vi "子VI-查看某框.vi"(0 "输入框号（默认值0为整张图）":dbl format="%#_13g", 1 "框组":T3(array[cluster]), 2 "临界Z值":i32, 3 "反射图原始路径":path, 4 "临界面积百分比值":dbl, 5 "预先配置的灰度阈值":dbl, 6 "穿透图原始路径":path, 7 "部位信息":string[](array[string])=["", "34.500000", "32.500000", "1121", "34", "54.955926", "分层类", "不合格", ""], 12 "产品规格":cluster{"产品长度（周长）（mm）":dbl, "产品宽度（母线长）（mm）":dbl}) -> (14 "全部检测结果":string[][](table))   [LabVIEW 2018]
uses:
  <vilib>/vision/NI_Vision_Development_Module.lvlib
panel:
  out "弥散类检测结果":string[][](table)
  out "?":string[][](table)
  in  "格式字符串 4":string="%f"
  in  "分隔符（'\\'代码显示） 3":string="\t"
  in  "返回主界面":bool caption="辅助定性分析"
  in  "格式字符串 3":string="%f"
  in  "分隔符（'\\'代码显示） 2":string="\t"
  out "弥散缺陷个数":i32
  out "分层缺陷个数":i32
  out "合格？ 弥散类":string="fencengThreshold"
  out "合格？分层类":string="fencengThreshold"
  in  "Tab Control":T1
  out "穿透ROI":T2(plugin-control)
  out "Threshold Image":T2(plugin-control)
  out "?":T2(plugin-control)
  out "?":T2(plugin-control)
  out "Threshold Image":T2(plugin-control)
  out "Threshold Image":T2(plugin-control)
  out "弥散测量结果":dbl[][](array[numeric]) format="%.2f"
  out "?":string
  out "面积 (pixels)":i32
  in  "格式字符串 2":string="%f"
  in  "分隔符（'\\'代码显示）":string="\t"
  out "分层测量结果":dbl[][](array[numeric]) format="%.2f"
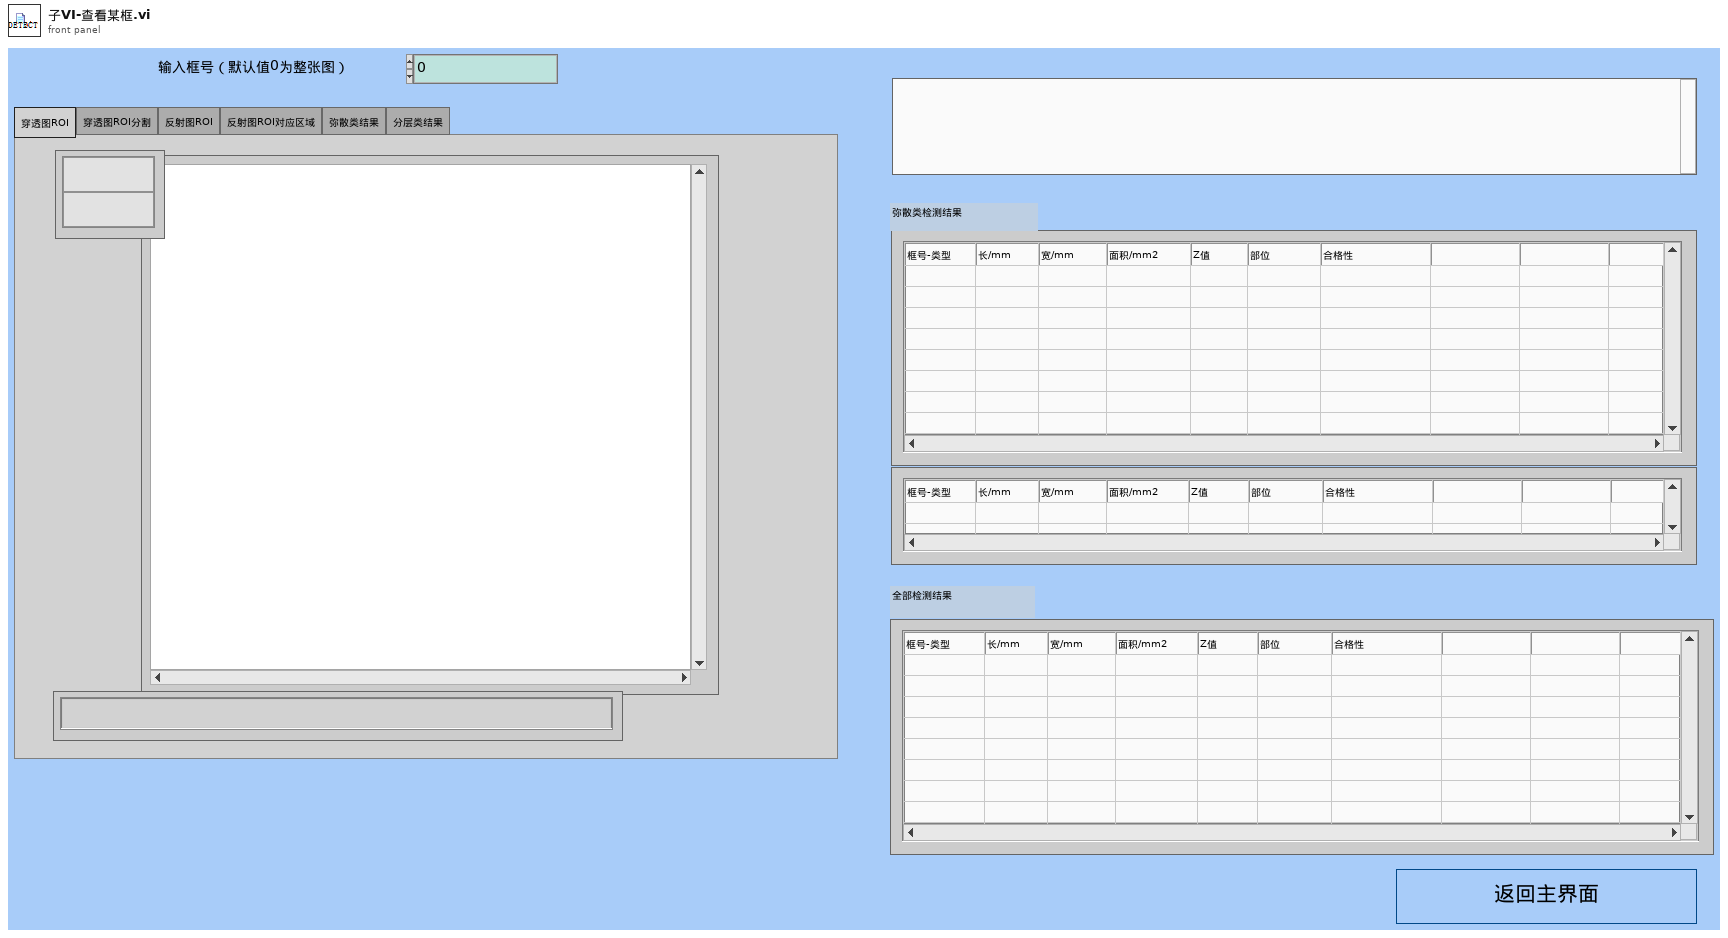
[diagram p1: front panel]
types:
  T1 = typedef "控件 1.ctl" = enum32{"穿透图ROI", "穿透图ROI分割", "反射图ROI", "反射图ROI对应区域", "弥散类结果", "分层类结果"}
  T2 = typedef "IMAQ Image.ctl" = refnum<image>
  T3 = cluster{"Global Rectangle":i32[], "Contours":cluster{"Contour Type":u32, "ROI Type":u32, "Points":i32[]}[]}[]
  T4 = cluster{"Zoom Tool":bool, "Selection Tool":bool, "Pan Tool":bool, "Point Tool":bool, "Line Tool":bool, "Rectangle Tool":bool, "Rotated Rectangle Tool":bool, "Polyline Tool":bool, "Polygon Tool":bool, "Freehand Tool":bool, "Closed Freehand Tool":bool, "Ellipse Tool":bool, "Annulus Tool":bool}
  T5 = typedef "Image Type" = u32
  T6 = typedef "Particle Parameters" = i32
  T7 = cluster{"Measurement Parameter":T6, "Range Lower Value":dbl, "Range Upper Value":dbl, "Range":bool, "Measurement Type":bool}[]
  T8 = cluster{"Global Rectangle":i32[], "Contours":cluster{"Contour Type":u32, "ROI Type":u32, "Points":i32[]}[]}
  T9 = cluster{"histogram":u32[], "Minimal Value":sgl, "Maximal Value":sgl, "Starting Value":sgl, "Interval Width":sgl, "Mean Value":sgl, "Standard  Variation":sgl, "Area (pixels)":i32}
  T10 = cluster{"Area":dbl, "Number of Holes":dbl, "Bounding Rect":cluster{"Left":dbl, "Top":dbl, "Right":dbl, "Bottom":dbl}, "Center of Mass":cluster{"X":dbl, "Y":dbl}, "Orientation":dbl, "Dimensions":cluster{"Width":dbl, "Height":dbl}}[]
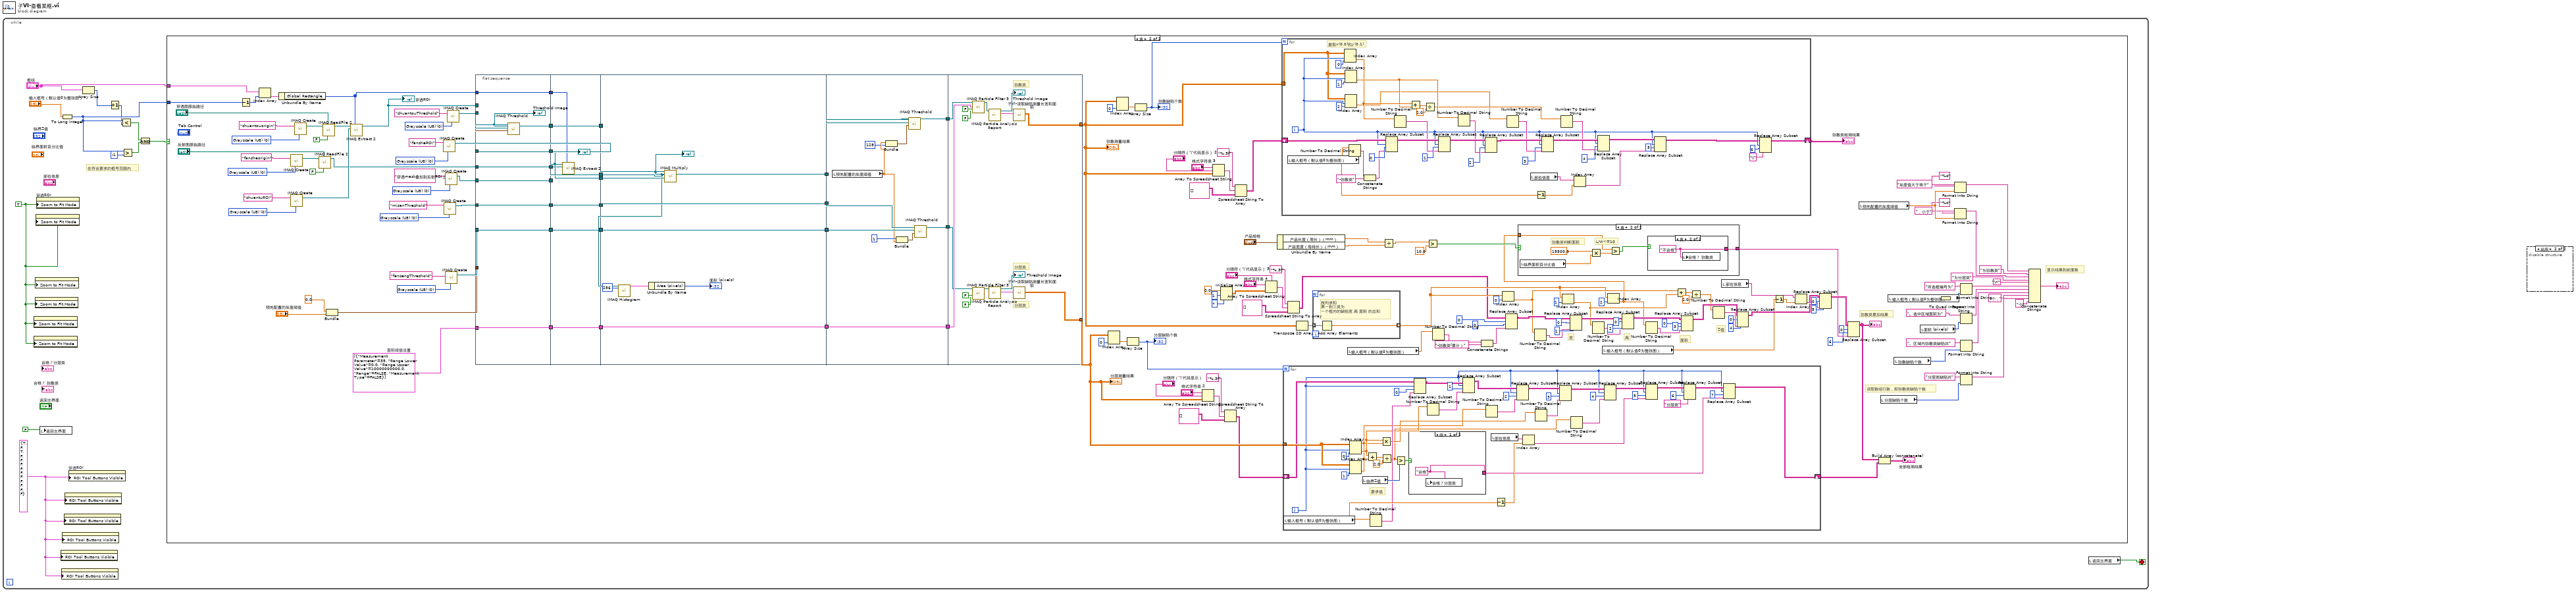
[diagram p0: block diagram]
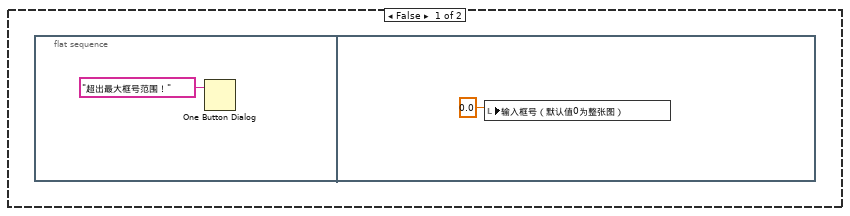
[diagram p2: hidden frame]
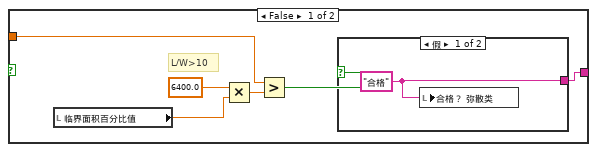
[diagram p3: hidden frame]
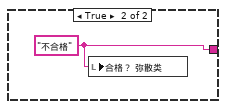
[diagram p4: hidden frame]
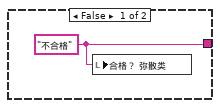
[diagram p5: hidden frame]
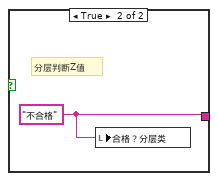
[diagram p6: hidden frame]
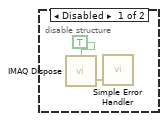
[diagram p7: hidden frame]
diagram:
  n1 = while {
    stop <- w5 stop-if-true
    w3 = T4 {"Zoom Tool"=TRUE, "Selection Tool"=FALSE, "Pan Tool"=TRUE, "Point Tool"=FALSE, "Line Tool"=FALSE, "Rectangle Tool"=FALSE, "Rotated Rectangle Tool"=FALSE, "Polyline Tool"=FALSE, "Polygon Tool"=FALSE, "Freehand Tool"=FALSE, "Closed Freehand Tool"=FALSE, "Ellipse Tool"=FALSE, "Annulus Tool"=FALSE} ("ROI Tool Buttons Visible:All Elements")
    w13 = TRUE ("Zoom to Fit Mode")
    # "在符合要求的框号范围内"
    n2 = property class="ImageControl"("Zoom to Fit Mode"=w13) -> ()  [unwired: 2 in, 2 out]
    n3 = property class="ImageControl"("Zoom to Fit Mode"=w13) -> ()  [unwired: 2 in, 2 out]
    n4 = property class="ImageControl"("Zoom to Fit Mode"=w13) -> ()  [unwired: 2 in, 2 out]
    n5 = property class="ImageControl"("Zoom to Fit Mode"=w13) -> ()  [unwired: 2 in, 2 out]
    n6 = property class="ImageControl"("Zoom to Fit Mode"=w13) -> ()  [unwired: 2 in, 2 out]
    n7 = property on="穿透ROI" class="ImageControl"("Zoom to Fit Mode"=w13) -> ()  [unwired: 2 in, 2 out]
    n8 = local write "返回主界面"(FALSE ("stop")) -> ()
    n9 = property class="ImageControl"("ROI Tool Buttons Visible"=w3) -> ()  [unwired: 2 in, 2 out]
    n10 = To Long Integer(number="输入框号（默认值0为整张图）") -> (32bit integer=w6:i32)
    n11 = property class="ImageControl"("ROI Tool Buttons Visible"=w3) -> ()  [unwired: 2 in, 2 out]
    n12 = property class="ImageControl"("ROI Tool Buttons Visible"=w3) -> ()  [unwired: 2 in, 2 out]
    n13 = property class="ImageControl"("ROI Tool Buttons Visible"=w3) -> ()  [unwired: 2 in, 2 out]
    n14 = property class="ImageControl"("ROI Tool Buttons Visible"=w3) -> ()  [unwired: 2 in, 2 out]
    n15 = property on="穿透ROI" class="ImageControl"("ROI Tool Buttons Visible"=w3) -> ()  [unwired: 2 in, 2 out]
    n16 = Array Size(array="框组") -> (size(s)=w2:i32)
    n17 = Increment(x=w2) -> (x+1=w1:i32)
    n18 = Less?(x=w6, y=w1) -> (x < y?=w11:bool)
    n19 = Greater?(x=w6, y=-1) -> (0:w10:bool)
    n20 = And(x=w11, y=w10) -> (x .and. y?=w4:bool)
    n21 = case shown="真" w4 {
      tunnel: "框组" -> [_ w77]
      tunnel: w6 -> [_ w76]
      frame False {
        n22 = flat-sequence {
          frame #0 {
            n23 = One Button Dialog(message="超出最大框号范围！" ("消息")) -> ()  [unwired: 1 in, 1 out]
          }
          frame #1 {
            n24 = local write "输入框号（默认值0为整张图）"(0.0 ("框号")) -> ()
          }
        }
      }
      frame True {
        w135 = T5 0 items=["Grayscale (U8)", "Grayscale (I16)", "Grayscale (SGL)", "Complex (CSG)", "RGB (U32)", "HSL (U32)", "RGB (U64)", "Grayscale (U16)"] ("Image Type")
        w136 = T5 0 items=["Grayscale (U8)", "Grayscale (I16)", "Grayscale (SGL)", "Complex (CSG)", "RGB (U32)", "HSL (U32)", "RGB (U64)", "Grayscale (U16)"] ("Image Type")
        w137 = T5 0 items=["Grayscale (U8)", "Grayscale (I16)", "Grayscale (SGL)", "Complex (CSG)", "RGB (U32)", "HSL (U32)", "RGB (U64)", "Grayscale (U16)"] ("Image Type")
        w141 = T5 0 items=["Grayscale (U8)", "Grayscale (I16)", "Grayscale (SGL)", "Complex (CSG)", "RGB (U32)", "HSL (U32)", "RGB (U64)", "Grayscale (U16)"] ("Image Type")
        w145 = T5 0 items=["Grayscale (U8)", "Grayscale (I16)", "Grayscale (SGL)", "Complex (CSG)", "RGB (U32)", "HSL (U32)", "RGB (U64)", "Grayscale (U16)"] ("Image Type")
        w120 = T7 [{"Measurement Parameter"=35, "Range Lower Value"=0.0, "Range Upper Value"=10000000000.0, "Range"=FALSE, "Measurement Type"=FALSE}]  # 面积阈值设置
        w156 = T5 0 items=["Grayscale (U8)", "Grayscale (I16)", "Grayscale (SGL)", "Complex (CSG)", "RGB (U32)", "HSL (U32)", "RGB (U64)", "Grayscale (U16)"] ("Image Type")
        w129 = T5 0 items=["Grayscale (U8)", "Grayscale (I16)", "Grayscale (SGL)", "Complex (CSG)", "RGB (U32)", "HSL (U32)", "RGB (U64)", "Grayscale (U16)"] ("Image Type")
        w160 = T5 0 items=["Grayscale (U8)", "Grayscale (I16)", "Grayscale (SGL)", "Complex (CSG)", "RGB (U32)", "HSL (U32)", "RGB (U64)", "Grayscale (U16)"] ("Image Type")
        # "弥散类累加结果"
        # "Z值"
        # "面积"
        # "高"
        # "宽"
        # "显示结果到前面板"
        # "读取数组行数，即弥散类缺陷个数"
        n25 = Decrement(x=w76) -> (x-1=w162:i32)
        n26 = Index Array(array=w77, index=w162) -> (element=w163:T8)
        n27 = Unbundle By Name(w163) -> ("Global Rectangle"=w128:i32[])
        n28 = call "IMAQ Create"("Image Name"="fansheorigin", "Image Type"=w141) -> ("New Image"=w140:T2)  [unwired: 3 in, 1 out]
        n29 = call "IMAQ Create"("Image Name"="chuantuROI", "Image Type"=w145) -> ("New Image"=w144:T2)  [unwired: 3 in, 1 out]
        n30 = call "IMAQ Create"("Image Name"="chuantouorigin", "Image Type"=w160) -> ("New Image"=w147:T2)  [unwired: 3 in, 1 out]
        n31 = call "IMAQ ReadFile 2"("Use File Path Image Type"=FALSE, "File Path"="反射图原始路径", "Image"=w140) -> ("Image Out"=w124:T2)  [unwired: 4 in, 4 out]
        n32 = call "IMAQ ReadFile 2"("Use File Path Image Type"=FALSE, "File Path"="穿透图原始路径", "Image"=w147) -> ("Image Out"=w148:T2)  [unwired: 4 in, 4 out]
        n33 = Bundle(0.0, "预先配置的灰度阈值"="预先配置的灰度阈值") -> (w119:cluster{dbl, "预先配置的灰度阈值":dbl})  [unwired: 1 in]
        n34 = call "IMAQ Extract 2"("Optional Rectangle"=w128, "Image Dst"=w144, "Image Src"=w148) -> ("Image Dst Out"=w126:T2)  [unwired: 7 in, 1 out]
        "穿透ROI" <- w126
        n35 = call "IMAQ Create"("Image Name"="fansheROI", "Image Type"=w129) -> ("New Image"=w125:T2)  [unwired: 3 in, 1 out]
        n36 = call "IMAQ Create"("Image Name"="misanThreshold", "Image Type"=w135) -> ("New Image"=w122:T2)  [unwired: 3 in, 1 out]
        n37 = call "IMAQ Create"("Image Name"="穿透mask叠加到反射ROI上", "Image Type"=w156) -> ("New Image"=w123:T2)  [unwired: 3 in, 1 out]
        n38 = call "IMAQ Create"("Image Name"="fencengThreshold", "Image Type"=w136) -> ("New Image"=w121:T2)  [unwired: 3 in, 1 out]
        n39 = call "IMAQ Create"("Image Name"="chuantouThreshold", "Image Type"=w137) -> ("New Image"=w127:T2)  [unwired: 3 in, 1 out]
        n40 = flat-sequence {
          tunnel: w128 -> [w257]
          tunnel: w127 -> [w256]
          tunnel: w126 -> [w255]
          tunnel: w119 -> [w254]
          tunnel: w125 -> [w253]
          tunnel: w124 -> [w252]
          tunnel: [w257] -> w186
          tunnel: [w253] -> w185
          tunnel: [w252] -> w184
          tunnel: [w251] -> w183
          tunnel: w123 -> [w251]
          tunnel: [w250] -> w182
          tunnel: w122 -> [w249]
          tunnel: [w249] -> w181
          tunnel: [w248] -> w180
          tunnel: w121 -> [w248]
          tunnel: [w247] -> w179
          tunnel: w120 -> [w247]
          tunnel: w186 -> [w266]
          tunnel: w185 -> [w258]
          tunnel: w184 -> [w259]
          tunnel: w183 -> [w265]
          tunnel: [w265] -> w178
          tunnel: [w264] -> w177
          tunnel: w182 -> [w264]
          tunnel: [w263] -> w176
          tunnel: w181 -> [w262]
          tunnel: [w262] -> w175
          tunnel: w180 -> [w261]
          tunnel: [w261] -> w174
          tunnel: w179 -> [w260]
          tunnel: [w260] -> w173
          tunnel: w178 -> [w276]
          tunnel: w177 -> [w275]
          tunnel: w176 -> [w274]
          tunnel: [w273] -> w172
          tunnel: w175 -> [w273]
          tunnel: w174 -> [w272]
          tunnel: [w272] -> w171
          tunnel: [w268] -> w170
          tunnel: w173 -> [w267]
          tunnel: [w267] -> w169
          tunnel: w172 -> [w287]
          tunnel: w171 -> [w286]
          tunnel: w170 -> [w285]
          tunnel: [w284] -> w168
          tunnel: [w283] -> w167
          tunnel: w169 -> [w282]
          tunnel: [w282] -> w166
          tunnel: [w291] -> w65
          tunnel: [w294] -> w108
          tunnel: w168 -> [w297]
          tunnel: w167 -> [w296]
          tunnel: w166 -> [w300]
          frame #0 {
            n41 = call "IMAQ Threshold"("Range"=w254, "Image Dst"=w256, "Image Src"=w255) -> ("Image Dst Out"=w250:T2)  [unwired: 3 in, 5 out]
            "Threshold Image" <- w250
          }
          frame #1 {
            n42 = call "IMAQ Extract 2"("Optional Rectangle"=w266, "Image Dst"=w258, "Image Src"=w259) -> ("Image Dst Out"=w263:T2)  [unwired: 7 in, 1 out]
            "?" <- w263
          }
          frame #2 {
            n43 = call "IMAQ Multiply"("Image Src A"=w275, "Image Dst"=w276, "Image Src B"=w274) -> ("Image Dst Out"=w268:T2)  [unwired: 4 in, 1 out]
            "?" <- w268
            n44 = call "IMAQ Histogram"("Number of Classes"=256, "Image"=w268) -> ("Histogram Report"=w270:T9)  [unwired: 8 in, 1 out]
            n45 = Unbundle By Name(w270) -> ("Area (pixels)"=→"面积 (pixels)":i32)
          }
          frame #3 {
            n46 = local read "预先配置的灰度阈值"() -> (w278:dbl)
            n47 = Bundle("预先配置的灰度阈值"=w278, 128) -> (w281:cluster{"预先配置的灰度阈值":dbl, i32})  [unwired: 1 in]
            n48 = Bundle(1, "预先配置的灰度阈值"=w278) -> (w280:cluster{i32, "预先配置的灰度阈值":dbl})  [unwired: 1 in]
            n49 = call "IMAQ Threshold"("Range"=w281, "Image Dst"=w287, "Image Src"=w285) -> ("Image Dst Out"=w283:T2)  [unwired: 3 in, 5 out]
            n50 = call "IMAQ Threshold"("Range"=w280, "Image Dst"=w286, "Image Src"=w285) -> ("Image Dst Out"=w284:T2)  [unwired: 3 in, 5 out]
          }
          frame #4 {
            # "分层类"
            # "分层类"
            # "弥散类"
            n51 = call "IMAQ Particle Filter 3"("Image Src"=w296, "Selection Values"=w300, "Keep/Remove Particles (F)"=FALSE, "Reject Border? (F)"=FALSE) -> ("Image Dst Out"=w289:T2)  [unwired: 9 in, 2 out]
            n52 = call "IMAQ Particle Filter 3"("Image Src"=w297, "Keep/Remove Particles (F)"=FALSE, "Reject Border? (F)"=FALSE) -> ("Image Dst Out"=w292:T2)  [unwired: 10 in, 2 out]
            n53 = call "IMAQ Particle Analysis Report"("Image"=w289) -> ("Particle Reports (Pixels)"=w290:T10, "Image Out (duplicate)"=→"Threshold Image":T2)  [unwired: 5 in, 4 out]
            n54 = call "IMAQ Particle Analysis Report"("Image"=w292) -> ("Particle Reports (Pixels)"=w295:T10, "Image Out (duplicate)"=→"Threshold Image":T2)  [unwired: 5 in, 4 out]
            n55 = call "子VI-读取缺陷测量长宽和面积.vi"("Particle Reports (Pixels)"=w290) -> ("测量结果"=w291:dbl[][])  [unwired: 10 in]
            n56 = call "子VI-读取缺陷测量长宽和面积.vi"("Particle Reports (Pixels)"=w295) -> ("测量结果"=w294:dbl[][])  [unwired: 10 in]
          }
        }
        n57 = Index Array(array=w108, index (col)=0 ("禁用的索引 (列)")) -> (element=w134:dbl[])  [unwired: 1 in]
        n58 = Index Array(array=w65, index (col)=0 ("禁用的索引 (列)")) -> (element=w132:dbl[])  [unwired: 1 in]
        n59 = Array Size(array=w134) -> (size(s)=w106:i32)
        "分层缺陷个数" <- w106
        n60 = Array Size(array=w132) -> (size(s)=w105:i32)
        "弥散缺陷个数" <- w105
        n61 = Array To Spreadsheet String(delimiter (Tab)="分隔符（'\\'代码显示）", array=w108, 3:"格式字符串 2") -> (spreadsheet string=w116:string)
        n62 = Array To Spreadsheet String(delimiter (Tab)="分隔符（'\\'代码显示） 2", array=w65, 3:"格式字符串 3") -> (spreadsheet string=w111:string)
        n63 = Initialize Array(0.0 ("元素"), 1 ("维数大小"), 7 ("维数大小")) -> (w66:dbl[][])
        n64 = Spreadsheet String To Array(format string="%.3f", spreadsheet string=w116, array type (2D Dbl)=string[][] [] ("Array")) -> (array=w107:string[][])  [unwired: 1 in]
        n65 = Spreadsheet String To Array(format string="%.3f", spreadsheet string=w111, array type (2D Dbl)=string[][] [] ("Array")) -> (array=w104:string[][])  [unwired: 1 in]
        n66 = Array To Spreadsheet String(delimiter (Tab)="分隔符（'\\'代码显示） 3", array=w66, 3:"格式字符串 4") -> (spreadsheet string=w69:string)
        n67 = Unbundle By Name("产品规格") -> ("产品长度（周长）（mm）"=w151:dbl, "产品宽度（母线长）（mm）"=w150:dbl)
        n68 = for {
          N: w105 -> [_]
          tunnel: w65 -> [w309]
          shift-right: [w325] -> w19
          shift-left: w104 -> [w331]
          i -> [w310]
          # "提取x(0,0)和y(0,1)"
          n69 = local read "输入框号（默认值0为整张图）"() -> (w313:dbl)
          n70 = Index Array(array=w309, index (row)=w310, index (col)=0 ("禁用的索引 (列)")) -> (element=w319:dbl)
          n71 = Index Array(array=w309, index (row)=w310, index (col)=2 ("索引 (列)")) -> (element=w308:dbl)
          n72 = Index Array(array=w309, index (row)=w310, index (col)=1 ("禁用的索引 (列)")) -> (element=w318:dbl)
          n73 = Number To Decimal String(number=w313) -> (decimal integer string=w305:string)  [unwired: 1 in]
          n74 = Concatenate Strings(w305, "-弥散类" ("新元素/子数组")) -> (w304:string)
          n75 = Replace Array Subset(array=w331, new element=w304, index (row)=w310, index (col)=0 ("索引 (列)")) -> (w330:string[][])
          n76 = Number To Decimal String(number=w319) -> (decimal integer string=w324:string)  [unwired: 1 in]
          n77 = Add(x=w319, y=w318) -> (x+y=w321:dbl)
          n78 = Divide(x=w321, y=2.0) -> (x/y=w317:dbl)
          n79 = Replace Array Subset(array=w330, new element=w324, index (row)=w310, index (col)=1 ("索引 (列)")) -> (w329:string[][])
          n80 = Number To Decimal String(number=w318) -> (decimal integer string=w323:string)  [unwired: 1 in]
          n81 = Replace Array Subset(array=w329, new element=w323, index (row)=w310, index (col)=2 ("索引 (列)")) -> (w328:string[][])
          n82 = Number To Decimal String(number=w308) -> (decimal integer string=w322:string)  [unwired: 1 in]
          n83 = local read "部位信息"() -> (w315:string[])
          n84 = Decrement(x=w313) -> (x-1=w314:dbl)
          n85 = Replace Array Subset(array=w328, new element=w322, index (row)=w310, index (col)=3 ("索引 (列)")) -> (w327:string[][])
          n86 = Number To Decimal String(number=w317) -> (decimal integer string=w316:string)  [unwired: 1 in]
          n87 = Index Array(array=w315, index=w314) -> (element=w312:string)
          n88 = Replace Array Subset(array=w327, new element=w316, index (row)=w310, index (col)=4 ("索引 (列)")) -> (w326:string[][])
          n89 = Replace Array Subset(array=w326, new element=w312, index (row)=w310, index (col)=5 ("索引 (列)")) -> (w307:string[][])
          n90 = Replace Array Subset(array=w307, new element="\\" ("新元素/子数组"), index (row)=w310, index (col)=6 ("索引 (列)")) -> (w325:string[][])
        }
        "弥散类检测结果" <- w19
        n91 = for {
          N: w106 -> [_]
          tunnel: w108 -> [w236]
          shift-right: [w214] -> w16
          shift-left: w107 -> [w225]
          i -> [w209]
          # "要求值"
          n92 = local read "输入框号（默认值0为整张图）"() -> (w234:dbl)
          n93 = Index Array(array=w236, index (row)=w209, index (col)=0 ("禁用的索引 (列)")) -> (element=w213:dbl)
          n94 = Index Array(array=w236, index (row)=w209, index (col)=1 ("禁用的索引 (列)")) -> (element=w212:dbl)
          n95 = local read "临界Z值"() -> (w242:i32)
          n96 = Add(x=w213, y=w212) -> (x+y=w243:dbl)
          n97 = Number To Decimal String(number=w234) -> (decimal integer string=w226:string)  [unwired: 1 in]
          n98 = Multiply(x=w213, y=w212) -> (x*y=w211:dbl)
          n99 = Divide(x=w243, y=2.0) -> (x/y=w208:dbl)
          n100 = Greater?(x=w208, y=w242) -> (0:w244:bool)
          n101 = case shown="假" w244 {
            tunnel: [w245 w246] -> w205
            frame False {
              w245 = "合格" ("合格？")
              n102 = local write "合格？分层类"(w245) -> ()
            }
            frame True {
              w246 = "不合格" ("合格？")
              # "分层判断Z值"
              n103 = local write "合格？分层类"(w246) -> ()
            }
          }
          n104 = Replace Array Subset(array=w225, new element=w226, index (row)=w209, index (col)=0 ("索引 (列)")) -> (w224:string[][])
          n105 = Number To Decimal String(number=w213) -> (decimal integer string=w223:string)  [unwired: 1 in]
          n106 = Replace Array Subset(array=w224, new element=w223, index (row)=w209, index (col)=1 ("索引 (列)")) -> (w221:string[][])
          n107 = Number To Decimal String(number=w212) -> (decimal integer string=w222:string)  [unwired: 1 in]
          n108 = local read "部位信息"() -> (w238:string[])
          n109 = Decrement(x=w234) -> (x-1=w237:dbl)
          n110 = Replace Array Subset(array=w221, new element=w222, index (row)=w209, index (col)=2 ("索引 (列)")) -> (w220:string[][])
          n111 = Index Array(array=w238, index=w237) -> (element=w207:string)
          n112 = Number To Decimal String(number=w211) -> (decimal integer string=w219:string)  [unwired: 1 in]
          n113 = Replace Array Subset(array=w220, new element=w219, index (row)=w209, index (col)=3 ("索引 (列)")) -> (w218:string[][])
          n114 = Number To Decimal String(number=w208) -> (decimal integer string=w210:string)  [unwired: 1 in]
          n115 = Replace Array Subset(array=w218, new element=w210, index (row)=w209, index (col)=4 ("索引 (列)")) -> (w217:string[][])
          n116 = Replace Array Subset(array=w217, new element=w207, index (row)=w209, index (col)=5 ("索引 (列)")) -> (w216:string[][])
          n117 = Replace Array Subset(array=w216, new element="分层类" ("新元素/子数组"), index (row)=w209, index (col)=6 ("索引 (列)")) -> (w215:string[][])
          n118 = Replace Array Subset(array=w215, new element=w205, index (row)=w209, index (col)=7 ("索引 (列)")) -> (w214:string[][])
        }
        n119 = Spreadsheet String To Array(format string="%.3f", spreadsheet string=w69, array type (2D Dbl)=string[][] [] ("Array")) -> (array=w38:string[][])  [unwired: 1 in]
        n120 = Transpose 2D Array(2D array=w65) -> (transposed array=w75:dbl[][])
        n121 = for {
          tunnel: w75 -> [w204] mode=indexing
          tunnel: [w203] -> w39 mode=indexing
          # "按列求和 \n第一到三类为\n一个框内的缺陷宽 高 面积 的总和"
          n122 = Add Array Elements(numeric array=w204) -> (sum=w203:dbl)
        }
        n123 = local read "输入框号（默认值0为整张图）"() -> (w40:dbl)
        n124 = Divide(x=w151, y=w150) -> (x/y=w154:dbl)
        n125 = Greater?(x=w154, y=10.0) -> (0:w26:bool)
        n126 = Number To Decimal String(number=w40) -> (decimal integer string=w43:string)  [unwired: 1 in]
        n127 = Concatenate Strings(w43, "-弥散类(累计）" ("新元素/子数组")) -> (w41:string)
        n128 = Index Array(array=w39, index=0 ("索引")) -> (element=w45:dbl)
        n129 = Replace Array Subset(array=w38, new element=w41, index (row)=0 ("禁用的索引 (行)"), index (col)=0 ("索引 (列)")) -> (w59:string[][])
        n130 = Number To Decimal String(number=w45) -> (decimal integer string=w58:string)  [unwired: 1 in]
        n131 = Index Array(array=w39, index=1 ("索引")) -> (element=w44:dbl)
        n132 = Replace Array Subset(array=w59, new element=w58, index (row)=0 ("索引 (行)"), index (col)=1 ("索引 (列)")) -> (w56:string[][])
        n133 = Number To Decimal String(number=w44) -> (decimal integer string=w49:string)  [unwired: 1 in]
        n134 = local read "输入框号（默认值0为整张图）"() -> (w22:dbl)
        n135 = Index Array(array=w39, index=2 ("索引")) -> (element=w25:dbl)
        n136 = case shown="真" w26 {
          tunnel: w25 -> [w190 w197]
          tunnel: [w187 w195] -> w20
          frame False {
            # "L/W>10"
            n137 = local read "临界面积百分比值"() -> (w189:dbl)
            n138 = Multiply(x=6400.0, y=w189) -> (x*y=w192:dbl)
            n139 = Greater?(x=w190, y=w192) -> (0:w188:bool)
            n140 = case shown="假" w188 {
              tunnel: [w193 w194] -> w187
              frame False {
                w193 = "合格" ("合格？")
                n141 = local write "合格？ 弥散类"(w193) -> ()
              }
              frame True {
                w194 = "不合格" ("合格？")
                n142 = local write "合格？ 弥散类"(w194) -> ()
              }
            }
          }
          frame True {
            # "弥散类判断面积"
            # "L/W<=10"
            n143 = local read "临界面积百分比值"() -> (w198:dbl)
            n144 = Multiply(x=15500.0, y=w198) -> (x*y=w199:dbl)
            n145 = Greater?(x=w197, y=w199) -> (0:w196:bool)
            n146 = case shown="真" w196 {
              tunnel: [w201 w202] -> w195
              frame False {
                w201 = "不合格" ("合格？")
                n147 = local write "合格？ 弥散类"(w201) -> ()
              }
              frame True {
                w202 = "不合格" ("合格？")
                n148 = local write "合格？ 弥散类"(w202) -> ()
              }
            }
          }
        }
        n149 = Replace Array Subset(array=w56, new element=w49, index (row)=0 ("索引 (行)"), index (col)=2 ("禁用的索引 (列)")) -> (w51:string[][])
        n150 = Number To Decimal String(number=w25) -> (decimal integer string=w48:string)  [unwired: 1 in]
        n151 = Add(x=w45, y=w44) -> (x+y=w47:dbl)
        n152 = Replace Array Subset(array=w51, new element=w48, index (row)=0 ("索引 (行)"), index (col)=3 ("索引 (列)")) -> (w34:string[][])
        n153 = Divide(x=w47, y=2.0) -> (x/y=w33:dbl)
        n154 = Number To Decimal String(number=w33) -> (decimal integer string=w37:string)  [unwired: 1 in]
        n155 = local read "部位信息"() -> (w28:string[])
        n156 = Replace Array Subset(array=w34, new element=w37, index (row)=0 ("索引 (行)"), index (col)=4 ("索引 (列)")) -> (w27:string[][])
        n157 = Decrement(x=w22) -> (x-1=w32:dbl)
        n158 = Index Array(array=w28, index=w32) -> (element=w31:string)
        n159 = Replace Array Subset(array=w27, new element=w31, index (row)=0 ("索引 (行)"), index (col)=5 ("索引 (列)")) -> (w21:string[][])
        n160 = Replace Array Subset(array=w21, new element=w20, index (row)=0 ("索引 (行)"), index (col)=6 ("索引 (列)")) -> (w17:string[][])
        "?" <- w17
        n161 = local read "预先配置的灰度阈值"() -> (w103:dbl)
        n162 = Build Array (concatenate)(w17, w16) -> (→"全部检测结果":string[][])
        n163 = local read "分层缺陷个数"() -> (w79:i32)
        n164 = local read "输入框号（默认值0为整张图）"() -> (w94:dbl)
        n165 = local read "弥散缺陷个数"() -> (w78:i32)
        n166 = local read "面积 (pixels)"() -> (w97:i32)
        n167 = To Quad Integer(1:w94) -> (0:w95:i64)
        n168 = Format Into String(format string="%d" ("格式字符串"), initial string="灰度值大于等于" ("初始字符串"), w103) -> (resulting string=w99:string)  [unwired: 1 in, 1 out]
        n169 = Format Into String(format string="%d" ("格式字符串"), initial string="，小于" ("初始字符串"), w103) -> (resulting string=w98:string)  [unwired: 1 in, 1 out]
        n170 = Format Into String(initial string="所选框编号为" ("初始字符串"), w95) -> (resulting string=w93:string)  [unwired: 2 in, 1 out]
        n171 = Format Into String(initial string="。选中区域面积为" ("字符串"), w97) -> (resulting string=w100:string)  [unwired: 2 in, 1 out]
        n172 = Format Into String(initial string="。区域内弥散类缺陷共" ("初始字符串"), w78) -> (resulting string=w101:string)  [unwired: 2 in, 1 out]
        n173 = Format Into String(initial string="分层类缺陷共" ("初始字符串"), w79) -> (resulting string=w102:string)  [unwired: 2 in, 1 out]
        n174 = Concatenate Strings(w99, "为弥散类" ("初始字符串"), w98, "为分层类" ("初始字符串"), "\n", w93, w100, w101, "个，" ("字符串"), w102, "个" ("字符串")) -> (→"?":string)
        "分层测量结果" <- w108
        "弥散测量结果" <- w65
      }
    }
    n175 = local read "返回主界面"() -> (w5:bool)
  }
  n176 = disable-structure shown="启用" {
    frame Disabled {
      n177 = call "IMAQ Dispose"("All Images? (No)"=TRUE) -> ("error out"=w342:errorcluster)  [unwired: 5 in]
      n178 = call <vilib>:"Simple Error Handler.vi"("error in (no error)"=w342) -> ()  [unwired: 4 in, 5 out]
    }
    frame Enabled {
    }
  }
